vi "SVT Convert FFT Spectrum to CPB Spectrum.vi"   [LabVIEW 2017, in "SoundVib_Octave.lvlib"]
uses:
  <vilib>/addons/Sound and Vibration/svt_Octave/SoundVib_Octave.lvlib
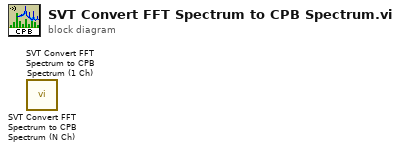
[diagram p0: block diagram]
diagram:
  n1 = call <vilib>:"SVT Convert FFT Spectrum to CPB Spectrum (N Ch).vi"() -> ()  [unwired: 15 in, 5 out]
  n2 = call <vilib>:"SVT Convert FFT Spectrum to CPB Spectrum (1 Ch).vi"() -> ()  [unwired: 15 in, 5 out]
